vi "Pre-Actor.vi"(8 "error in":errorcluster, 11 "ProXR in":refnum<class "ProXR.lvclass">) -> (0 "error out":errorcluster, 3 "ProXR out":refnum<class "ProXR.lvclass">)   [LabVIEW 2019, in "ProXR.lvlib" / "ProXR.lvclass"]
doc: "This override VI is to provide the means for children classes to perform application specific post launch initialization functions that must be performed *prior* to calling the actor. \n\n***DO NOT USE THE CHECK FOR FAULT ROUTINE HERE***"
uses:
  Library/ProXR.lvclass
  builds/Instruments/DIG_IO.lvlibp/Library/DIG_IO.lvclass
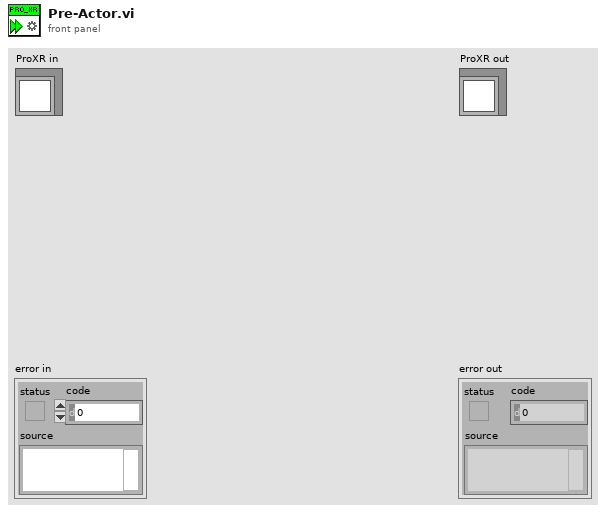
[diagram p1: front panel]
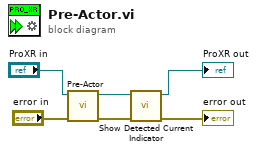
[diagram p0: block diagram]
diagram:
  n1 = call-parent "Pre-Actor.vi"("error in"="error in", "DIG_IO in"="ProXR in") -> ("error out"=w3:errorcluster, "DIG_IO out"=w4:refnum<class "ProXR.lvclass">)  [unwired: 8 in]
  n2 = call "Show Detected Current Indicator.vi"("error in"=w3, "ProXR in"=w4) -> ("error out"=→"error out":errorcluster, "ProXR out"=→"ProXR out":refnum<class "ProXR.lvclass">)  [unwired: 8 in]
